vi "Motion Profile Tester.vi"() -> ()   [LabVIEW 2015]
uses:
  <vilib>/Rock Robotics/WPI/CAN/TalonSRX/WPI_CANTalonSRX_MotionProfileTrajectoryPt.ctl
  <vilib>/Rock Robotics/WPI/CAN/TalonSRX/WPI_CANTalonSRX_APIControlMode.ctl
  <vilib>/Rock Robotics/WPI/CAN/TalonSRX/WPI_CANTalonSRX_APIFeedbackSelect.ctl
  Support Code/Team900-VIs/OnButton/OnButtonSingle.vi
  <vilib>/Rock Robotics/WPI/MotorControl/WPI_MotorControlOpenCANTalonSRX.vi
panel:
  out "Motor values while Running Profile":cluster{dbl[], dbl[]}[](graph)
  out "Applied Throttle while Running Profile":cluster{dbl[], dbl[]}(graph)
  in  "Run at 100% Power and Graph":bool
  in  "Abort":bool
  in  "Generate, Load, and Run Profile":bool
  in  "Run Profile":bool
  in  "Load Profile":bool
  in  "Generate Profile and Clear Points":bool
  out "Generated Profile":cluster{dbl[], dbl[]}[](graph)
  in  "Mode":T1(ring)
  in  "Motion Profile Control Frame Rate":dbl
  in  "Rotations to Travel":dbl
  in  "Max Jerk (rotations/sec^3)":dbl
  in  "Max Acceleration (rotations/sec^2)":dbl
  in  "Max Speed (rotations/sec)":dbl
  # "If applied throttle exceeds about .95 at any point in the execution of the profile either max speed acceleration, or jerk must be lowered. If it goes below .8 except at the very beginning or end either max speed, acceleration, or jerk  should be increased. (These numbers are for profiles which are supposed to be completed as quickly as possible. In contexts where the priority is on other things such as reducing the amount of force or jerk acting on a gearbox other metrics must be used.)"
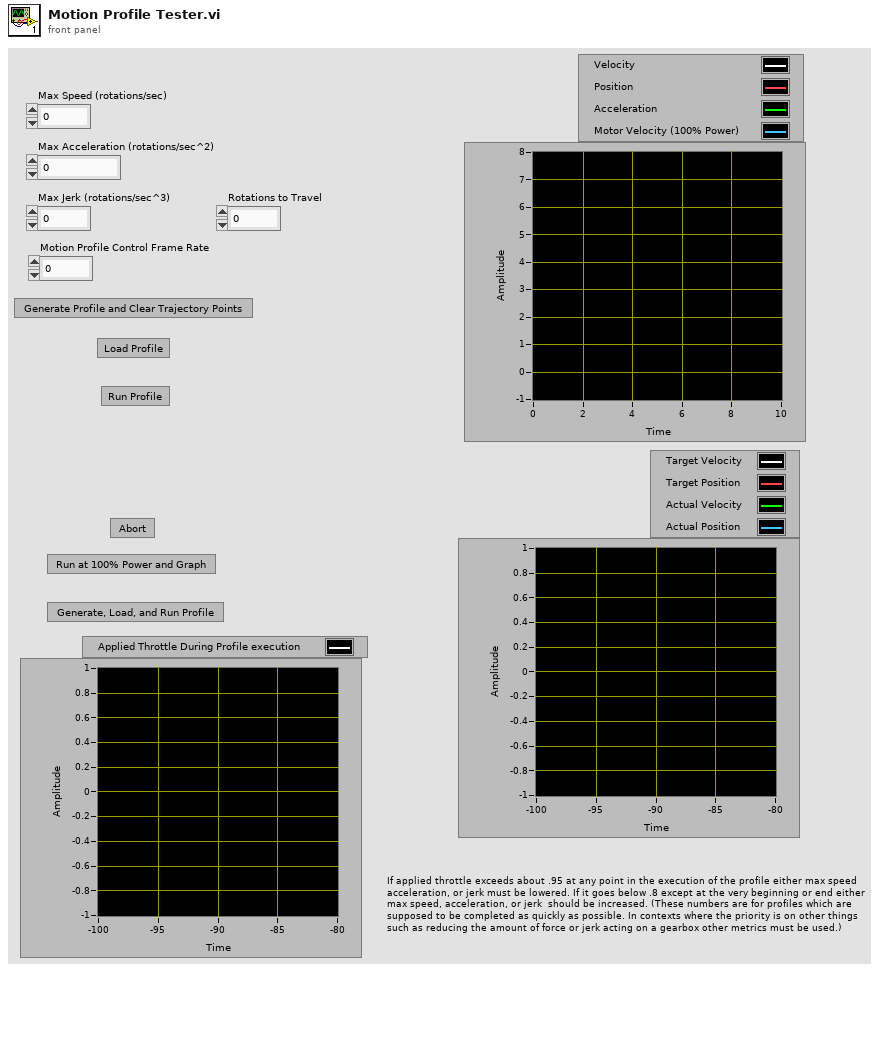
[diagram p1: front panel]
types:
  T1 = enum16{"Nothing", "Generate Profile and Clear", "Load Data to Motor", "Run Profile", "Run at 100% power and log"}
  T2 = typedef "WPI_CANTalonSRX_APIFeedbackSelect.ctl" = enum16{"Digital Quadrature Encoder", "Analog Potentiometer", "Analog Encoder", "Count on Quad-A (Rising-Edge)", "Count on Quad-A (Falling-Edge)", "CTR Magnetic Enc (Absolute)", "CTR Magnetic Enc (Relative)", "Pulse Width"}
  T3 = typedef "WPI_CANTalonSRX_APIControlMode.ctl" = enum8{"Percent VBus", "Speed", "Position", "Slave", "Unchanged / Invalid", "Voltage Compensation", "Current", "Motion Profile"}
  T4 = typedef "WPI_MotorControlDeviceRef.ctl" = cluster{"DeviceStatus":errorcluster, "Type":T5, "PWM":cluster{"PWM Channel":T6, "DeadBand":T7}, "CAN":cluster{"Device Number":u8, "Control Mode":T8, "Semaphore":T9, "Max Vout":dbl, "TalonSRX Control Mode":T3}, "Invert":bool}
  T5 = typedef "WPI_MotorControlType.ctl" = enum16{"PWM", "CAN", "CANTalonSRX"}
  T6 = typedef "FPGA_DIOPWMChannel.ctl" = enum8{"PWM 0", "PWM 1", "PWM 2", "PWM 3", "PWM 4", "PWM 5", "PWM 6", "PWM 7", "PWM 8", "PWM 9", "PWM MXP 0", "PWM MXP 1", "PWM MXP 2", "PWM MXP 3", "PWM MXP 4", "PWM MXP 5", "PWM MXP 6", "PWM MXP 7", "PWM MXP 8", "PWM MXP 9", "Invalid"}
  T7 = typedef "WPI_PWMDeadband.ctl" = cluster{"Name":string, "maxPositivePwm":i32, "minPositivePwm":i32, "centerPwm":i32, "maxNegativePwm":i32, "minNegativePwm":i32, "angularRange":u16}
  T8 = typedef "WPI_CANJaguar_ControlMode.ctl" = enum8{"Percent VBus", "Current", "Speed", "Position", "Voltage"}
  T9 = typedef "Semaphore RefNum" = refnum<k1>
  T10 = typedef "WPI_CANTalonSRX_MotionProfileTrajectoryPt.ctl" = cluster{"Duration Ms":u8, "Velocity":dbl, "Position":dbl, "Profile Slot Select":u8, "Is Last":bool, "Velocity Only":bool, "Zero Position":bool, "Compress Code":u8, "Same Velocity":i32, "Delta Position":i32, "Count":u8}
  T11 = enum16{"Nothing", "Generate Profile and Clear", "Load Data to Motor", "Run Profile"}
  T12 = enum16{"Nothing", "Generate Profile and Clear", "Load Data to Motor", "Run Profile", "Run at 100% power and log"}[]
  T13 = typedef "WPI_CANTalonSRX_GlobalStatus.ctl" = cluster{"Applied Throttle":dbl, "Module Enabled":bool, "CAN Error":errorcluster, "Closed Loop Error":dbl, "Forward Limit Switch Closed":bool, "Reverse Limit Switch Closed":bool, "Sensor Position":dbl, "Sensor Velocity":dbl, "Current":dbl, "Sticky Fault - Over Temp":bool, "Sticky Fault - Under Voltage":bool, "Sticky Fault - Forward Limit":bool, "Sticky Fault - Reverse Limit":bool, "Sticky Fault - Forward Soft Limit":bool, "Sticky Fault - Reverse Soft Limit":bool, "Brake is Enabled":bool, "Encoder Position":dbl, "Encoder Velocity":dbl, "Encoder Index Count":dbl, "Encoder A Pin State":bool, "Encoder B Pin State":bool, "Encoder Index Pin State":bool, "Analog In":dbl, "Analog In Velocity":dbl, "Temperature (C)":dbl, "Battery Voltage":dbl, "Control 5 Is Supported":bool, "Current Profile Slot Select":dbl, "Pos Div 8":bool, "Vel Div 4":bool, "Pulse Width Position":i32, "Pulse Width Velocity":i32, "Pulse Width Rise To Rise (us)":i32, "Pulse Width Rise To Fall (us)":i32, "Mot Prof Active Is Under Run":bool, "Mot Prof Active Has Under Run":bool, "Mot Prof Active Is Last":bool, "Mot Prof Active Velocity Only":bool, "Mot Prof Active Is Valid":bool, "Mot Prof Buffer Is Full":bool, "Mot Prof Active Profile Slot Select":i32, "Mot Prof NextID":i32, "Mot Prof Count":i32, "Mot Prof Active Velocity":dbl, "Mot Prof Active Position":dbl, "Mot Prof Output Enable":i32}
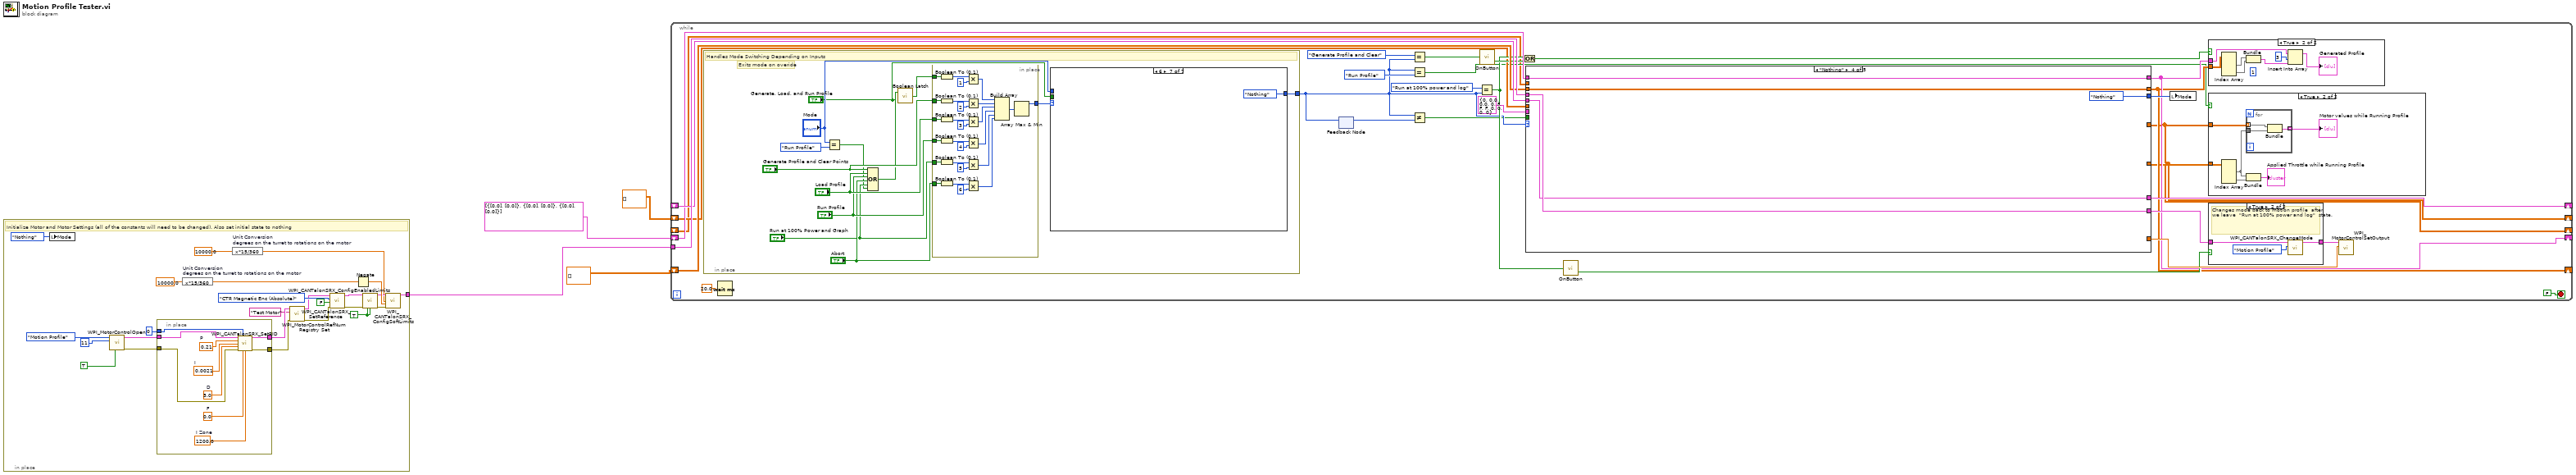
[diagram p0: block diagram]
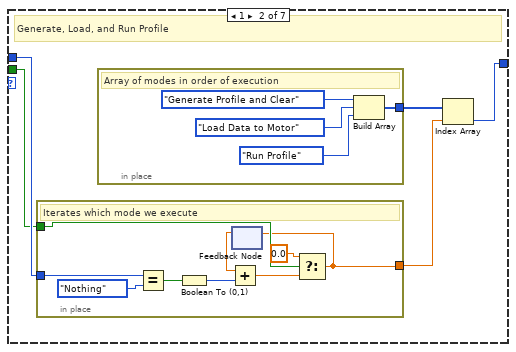
[diagram p6: hidden frame]
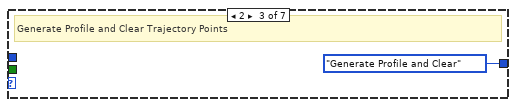
[diagram p7: hidden frame]
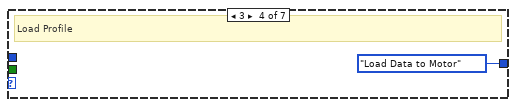
[diagram p8: hidden frame]
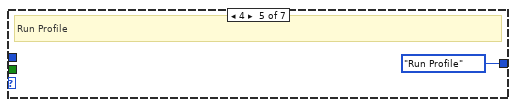
[diagram p9: hidden frame]
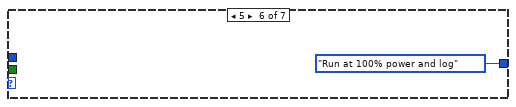
[diagram p10: hidden frame]
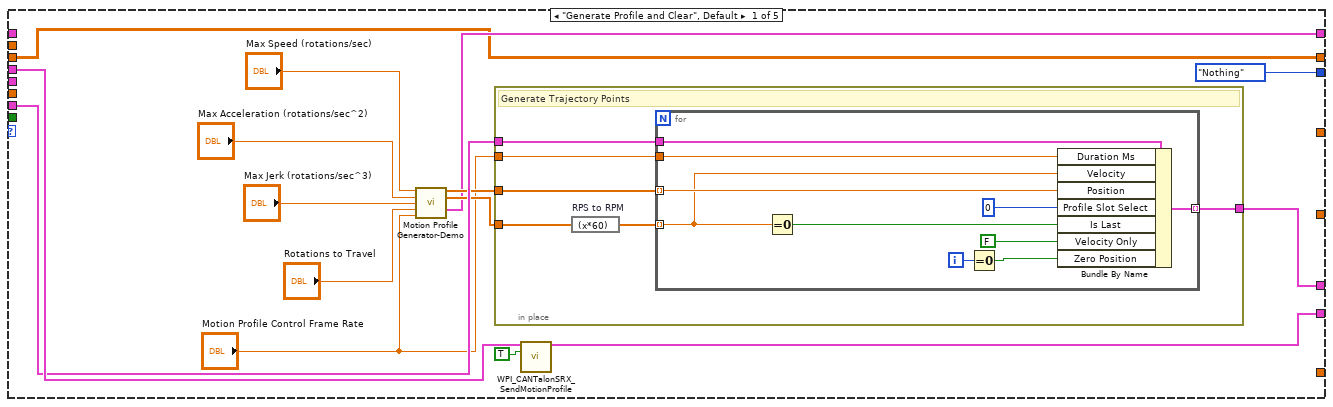
[diagram p11: hidden frame]
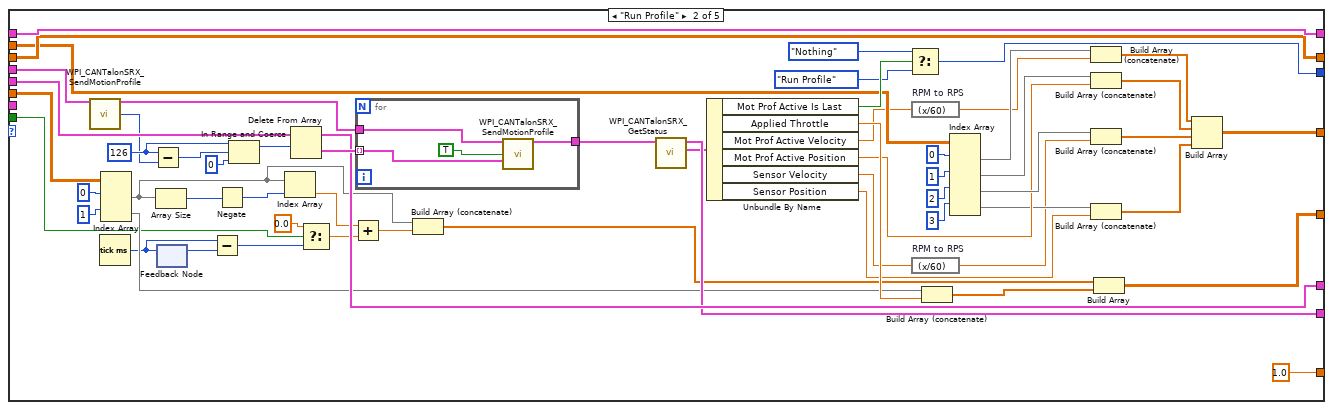
[diagram p12: hidden frame]
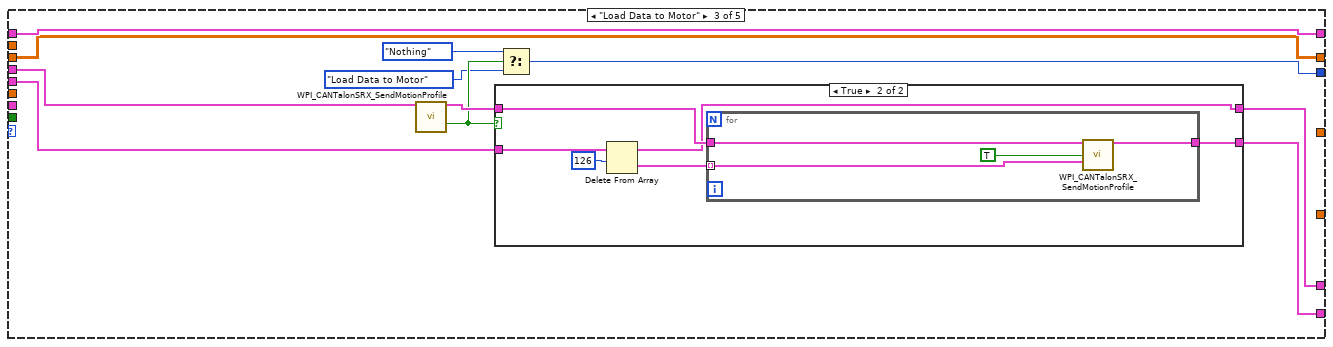
[diagram p13: hidden frame]
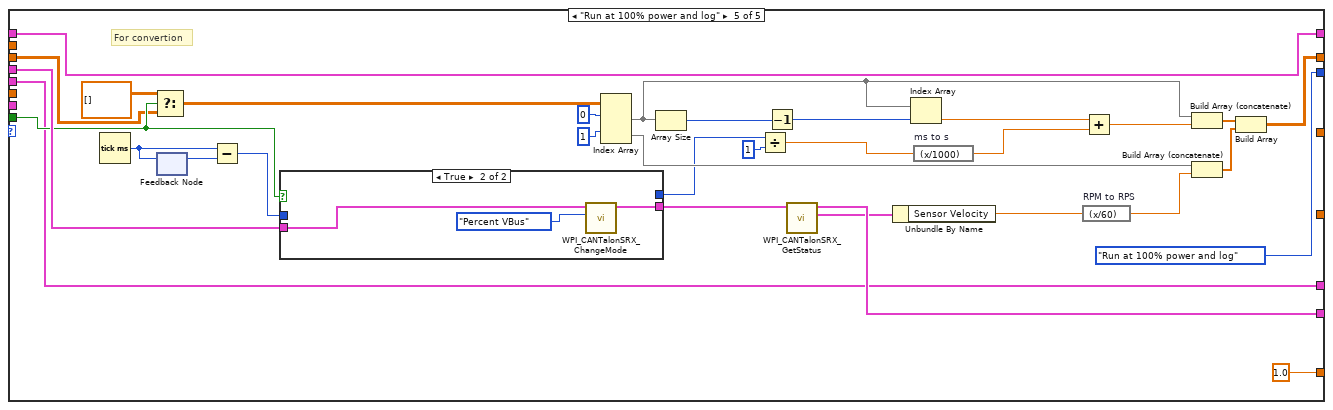
[diagram p15: hidden frame]
diagram:
  n1 = in-place {
    in-place-border: [w23] -> w4
    w19 = TRUE ("Forward Soft Limit Enable")
    # "Initialize Motor and Motor Settings (all of the constants will need to be changed). Also set initial state to nothing"
    n2 = local write "Mode"(T1."Nothing" ("Mode")) -> ()
    n3 = call-poly <vilib>:"WPI_MotorControlOpen.vi"("Invert"=TRUE, "Device Number"=11, "Control Mode"=WPI_CANTalonSRX_APIControlMode."Motion Profile") -> ("error out"=w26:errorcluster, "MotorControlDeviceRef"=w27:T4)  [unwired: 7 in]
    n4 = in-place {
      in-place-border: w27 -> [w39]
      in-place-border: w26 -> [w38]
      in-place-border: [w30] -> w10
      in-place-border: [w31] -> w12
      in-place-border: u8 0 ("Parameter Slot") -> [w32]
      w33 = 1200.0  # I Zone
      w34 = 0.0  # F
      w35 = 3.0  # D
      w36 = 0.0021  # I
      w37 = 0.21  # P
      n5 = call <vilib>:"WPI_CANTalonSRX_SetPID.vi"("CAN Talon SRX Ref"=w39, "Parameter Slot"=w32, "P"=w37, "I"=w36, "D"=w35, "error in (no error)"=w38, "F"=w34, "I Zone"=w33) -> ("CAN Talon SRX Ref"=w31:T4, "error out"=w30:errorcluster)  [unwired: 6 in]
    }
    n6 = expression code="x*15/360" "Unit Conversion\ndegrees on the turret to rotations on the motor"(10000.0 ("Forward Limit Position")) -> (w21:dbl)
    n7 = expression code="x*15/360" "Unit Conversion\ndegrees on the turret to rotations on the motor"(10000.0 ("Forward Limit Position")) -> (w13:dbl)
    n8 = call <vilib>:"WPI_MotorControlRefNum Registry Set.vi"("error in (no error)"=w10, "refnum name"="Test Motor", "MotorControlDevRef"=w12) -> ("error out"=w9:errorcluster, "MotorControlDevRef"=w11:T4)  [unwired: 7 in]
    n9 = call <vilib>:"WPI_CANTalonSRX_SetReference.vi"("error in (no error)"=w9, "Reverse Feedback Sensor"=FALSE, "Feedback Reference"=WPI_CANTalonSRX_APIFeedbackSelect."CTR Magnetic Enc (Absolute)", "CAN Talon SRX Ref"=w11) -> ("error out"=w6:errorcluster, "CAN Talon SRX Ref"=w7:T4)  [unwired: 6 in]
    n10 = Negate(x=w21) -> (-x=w20:dbl)
    n11 = call <vilib>:"WPI_CANTalonSRX_ConfigEnabledLimits.vi"("CAN Talon SRX Ref"=w7, "error in (no error)"=w6, "Forward Soft Limit Enable"=w19, "Reverse Soft Limit Enable"=w19) -> ("CAN Talon SRX Ref"=w17:T4, "error out"=w18:errorcluster)  [unwired: 10 in]
    n12 = call <vilib>:"WPI_CANTalonSRX_ConfigSoftLimits.vi"("CAN Talon SRX Ref"=w17, "Forward Limit Position"=w13, "Reverse Limit Position"=w20, "error in (no error)"=w18) -> ("CAN Talon SRX Ref"=w23:T4)  [unwired: 10 in, 1 out]
  }
  n13 = while {
    tunnel: w4 -> [w69]
    shift-right: [w67] -> _
    shift-left: _ -> [w64]
    shift-right: [w54] -> _
    shift-left: cluster{dbl[], dbl[]}[] [{[0.0], [0.0]}, {[0.0], [0.0]}, {[0.0], [0.0]}] ("XY Graph") -> [w56]
    shift-right: [w53] -> _
    shift-left: dbl[][] [] -> [w55]
    shift-right: [w45] -> _
    shift-left: dbl[][] [] -> [w48]
    shift-right: [w43] -> _
    shift-left: _ -> [w44]
    stop <- FALSE stop-if-true
    n14 = in-place {
      in-place-border: [w101] -> w42
      # "Exits mode on overide"
      # "Handles Mode Switching Depending on Inputs"
      n15 = Equal?(x="Mode", y=T11."Run Profile") -> (x = y?=w92:bool)
      n16 = Compound Arithmetic op=OR("Generate Profile and Clear Points", "Load Profile", "Run Profile", "Abort", "Run at 100% Power and Graph", w92) -> (w91:bool)
      n17 = call "Boolean Latch.vi"("Input"="Generate, Load, and Run Profile", "Reset"=w91) -> ("Output"=w98:bool)
      n18 = in-place {
        in-place-border: "Generate Profile and Clear Points" -> [w128]
        in-place-border: "Load Profile" -> [w123]
        in-place-border: w98 -> [w121]
        in-place-border: "Run Profile" -> [w119]
        in-place-border: [w117] -> w99
        in-place-border: "Abort" -> [w108]
        in-place-border: "Run at 100% Power and Graph" -> [w105]
        n19 = Boolean To (0,1)(Boolean=w121) -> (0, 1=w115:i16)
        n20 = Boolean To (0,1)(Boolean=w128) -> (0, 1=w127:i16)
        n21 = Boolean To (0,1)(Boolean=w123) -> (0, 1=w125:i16)
        n22 = Boolean To (0,1)(Boolean=w119) -> (0, 1=w116:i16)
        n23 = Boolean To (0,1)(Boolean=w105) -> (0, 1=w104:i16)
        n24 = Boolean To (0,1)(Boolean=w108) -> (0, 1=w107:i16)
        n25 = Multiply(x=w115, y=i16 1) -> (x*y=w112:i16)
        n26 = Multiply(x=w127, y=i16 2) -> (x*y=w111:i16)
        n27 = Multiply(x=w125, y=i16 3) -> (x*y=w110:i16)
        n28 = Multiply(x=w116, y=i16 4) -> (x*y=w109:i16)
        n29 = Multiply(x=w104, y=i16 5) -> (x*y=w103:i16)
        n30 = Multiply(x=w107, y=i16 6) -> (x*y=w106:i16)
        n31 = Build Array(w112, w111, w110, w109, w103, w106) -> (w118:i16[])
        n32 = Array Max & Min(array=w118) -> (max value=w117:i16)  [unwired: 3 out]
      }
      n33 = case shown="6" w99 {
        tunnel: [w129 w130 T1."Generate Profile and Clear" ("Mode") T1."Load Data to Motor" ("Mode") T1."Run Profile" ("Mode") T1."Run at 100% power and log" ("Mode") T1."Nothing" ("Mode")] -> w101
        tunnel: "Mode" -> [w129 w134 _ _ _ _ _]
        tunnel: "Generate, Load, and Run Profile" -> [_ w133 _ _ _ _ _]
        frame 0, Default {
          # "Carry last operation"
        }
        frame 1 {
          # "Generate, Load, and Run Profile"
          n34 = in-place {
            in-place-border: w134 -> [w143]
            in-place-border: w133 -> [w138]
            in-place-border: [w135] -> w131
            # "Iterates which mode we execute"
            n35 = Equal?(x=w143, y=T11."Nothing") -> (x = y?=w141:bool)
            n36 = Boolean To (0,1)(Boolean=w141) -> (0, 1=w140:i16)
            n37 = feedback #1() -> (w139:dbl)  [unwired: 1 in]
            n38 = Add(x=w139, y=w140) -> (x+y=w136:dbl)
            n39 = Select(t=0.0, s=w138, f=w136) -> (s? t:f=w135:dbl)
            n40 = feedback-in #1(w135) -> ()
          }
          n41 = in-place {
            in-place-border: [w147] -> w132
            # "Array of modes in order of execution"
            n42 = Build Array(T1."Generate Profile and Clear" ("Mode"), T1."Load Data to Motor" ("Mode"), T1."Run Profile" ("Mode")) -> (w147:T12)
          }
          n43 = Index Array(array=w132, index=w131) -> (element=w130:T1)
        }
        frame 2 {
          # "Generate Profile and Clear Trajectory Points"
        }
        frame 3 {
          # "Load Profile"
        }
        frame 4 {
          # "Run Profile"
        }
        frame 5 {
        }
        frame 6 {
        }
      }
    }
    n44 = Wait (ms)(milliseconds to wait=20.0) -> ()  [unwired: 1 out]
    n45 = feedback-in #2(w42) -> ()
    n46 = feedback #2() -> (w41:T1)  [unwired: 1 in]
    n47 = Equal?(x=T1."Generate Profile and Clear", y=w42) -> (x = y?=w52:bool)
    n48 = Equal?(x=w42, y=T1."Run Profile") -> (x = y?=w46:bool)
    n49 = Not Equal?(x=w42, y=w41) -> (x != y?=w40:bool)
    n50 = Equal?(x=T1."Run at 100% power and log", y=w42) -> (x = y?=w49:bool)
    n51 = call-poly "OnButton.vi"("Input"=w52) -> ("Released"=w51:bool)  [unwired: 1 out]
    n52 = Or(x=w49, y=w51) -> (x .or. y?=w50:bool)
    n53 = case shown="\"Nothing\"" w42 {
      tunnel: w69 -> [w163 w240 w256 w274 w306]
      tunnel: T10 {"Duration Ms"=0, "Velocity"=0.0, "Position"=0.0, "Profile Slot Select"=0, "Is Last"=FALSE, "Velocity Only"=FALSE, "Zero Position"=FALSE, "Compress Code"=0, "Same Velocity"=0, "Delta Position"=0, "Count"=0} ("New Point") -> [w162 _ _ _ _]
      tunnel: [w159 w234 w254 w273 w276] -> w67
      tunnel: [T1."Nothing" ("Mode") w231 w252 T1."Nothing" ("Mode") T1."Run at 100% power and log" ("Mode")] -> w65
      tunnel: w64 -> [_ w241 w257 w273 w276]
      tunnel: [w158 w233 w251 w274 w302] -> w58
      tunnel: [_ 1.0 _ _ 1.0] -> w62
      tunnel: w40 -> [_ w195 _ _ w293]
      tunnel: [w155 w224 w247 w270 w295] -> w53
      tunnel: [w156 w225 w248 w271 w301] -> w54
      tunnel: w56 -> [_ w225 w248 w271 w301]
      tunnel: w55 -> [w155 w224 w247 w270 w292]
      tunnel: w48 -> [_ w223 _ _ _]
      tunnel: [_ w219 _ _ _] -> w45
      tunnel: w44 -> [_ w211 _ _ _]
      tunnel: [_ w198 _ _ _] -> w43
      frame "Generate Profile and Clear", Default {
        n54 = call "Motion Profile Generator-Demo.vi"("Max Speed (rotations/sec)"="Max Speed (rotations/sec)", "Max Acceleration (rotations/sec^2)"="Max Acceleration (rotations/sec^2)", "Max Jerk (rotations/sec^3)"="Max Jerk (rotations/sec^3)", "Rotations to Travel"="Rotations to Travel", "Motion Profile Control Frame Rate"="Motion Profile Control Frame Rate") -> ("Position rotations"=w160:dbl[], "velocity rotations/sec"=w161:dbl[], "XY Graph"=w156:cluster{dbl[], dbl[]}[])  [unwired: 7 in, 1 out]
        n55 = in-place {
          in-place-border: w162 -> [w173]
          in-place-border: w161 -> [w169]
          in-place-border: w160 -> [w172]
          in-place-border: "Motion Profile Control Frame Rate" -> [w171]
          in-place-border: [w170] -> w159
          # "Generate Trajectory Points"
          n56 = expression code="(x*60)" "RPS to RPM"(w169) -> (w168:dbl[])
          n57 = for {
            tunnel: w173 -> [w183]
            tunnel: w168 -> [w179] mode=indexing
            tunnel: w172 -> [w181] mode=indexing
            tunnel: w171 -> [w180]
            tunnel: [w174] -> w170 mode=indexing
            i -> [w176]
            n58 = Equal To 0?(x=w179) -> (x = 0?=w178:bool)
            n59 = Equal To 0?(x=w176) -> (x = 0?=w175:bool)
            n60 = Bundle By Name(cluster=w183, "Duration Ms"=w180, "Velocity"=w179, "Position"=w181, "Profile Slot Select"=u8 0, "Is Last"=w178, "Velocity Only"=FALSE, "Zero Position"=w175) -> (w174:T10)
          }
        }
        n61 = call <vilib>:"WPI_CANTalonSRX_SendMotionProfile.vi"("CAN Talon SRX Ref"=w163, "Clear"=TRUE) -> ("CAN Talon SRX Ref Out"=w158:T4)  [unwired: 10 in, 3 out]
      }
      frame "Run Profile" {
        w238 = u32 126 ("x")
        n62 = call <vilib>:"WPI_CANTalonSRX_SendMotionProfile.vi"("CAN Talon SRX Ref"=w240) -> ("CAN Talon SRX Ref Out"=w228:T4, "Count"=w229:u32)  [unwired: 11 in, 2 out]
        n63 = Tick Count (ms)() -> (millisecond timer value=w197:u32)
        n64 = Index Array(array=w223, index (row) #1=0 ("index (row)"), index (row) #2=1 ("index (row)")) -> (element #1=w190:dbl[], element #2=w221:dbl[])  [unwired: 2 in]
        n65 = Subtract(x=w238, y=w229) -> (x-y=w239:u32)
        n66 = Array Size(array=w190) -> (size(s)=w192:i32)
        n67 = feedback #3() -> (w196:u32)  [unwired: 1 in]
        n68 = feedback-in #3(w197) -> ()
        n69 = Subtract(x=w197, y=w196) -> (x-y=w193:u32)
        n70 = Negate(x=w192) -> (-x=w191:i32)
        n71 = In Range and Coerce(upper limit=w238, x=w239, lower limit=u32 0) -> (coerced(x)=w235:u32)  [unwired: 1 out]
        n72 = Index Array(array=w190, index=w191) -> (element=w189:dbl)
        n73 = Delete From Array(array=w241, length=w235) -> (deleted portion=w236:T10[], array with subset deleted=w234:T10[])  [unwired: 1 in]
        n74 = Select(t=0.0, s=w195, f=w193) -> (s? t:f=w188:dbl)
        n75 = Add(x=w189, y=w188) -> (x+y=w220:dbl)
        n76 = for {
          tunnel: w236 -> [w246] mode=indexing
          tunnel: w228 -> [w244]
          tunnel: [w243] -> w216
          n77 = call <vilib>:"WPI_CANTalonSRX_SendMotionProfile.vi"("CAN Talon SRX Ref"=w244, "Push"=TRUE, "New Point"=w246) -> ("CAN Talon SRX Ref Out"=w243:T4)  [unwired: 9 in, 3 out]
        }
        n78 = Build Array (concatenate)(w190, w220) -> (w218:dbl[])
        n79 = call <vilib>:"WPI_CANTalonSRX_GetStatus.vi"("CAN Talon SRX Ref"=w216) -> ("Talon SRX Status"=w232:T13, "CAN Talon SRX Ref"=w233:T4)  [unwired: 8 in, 1 out]
        n80 = Unbundle By Name(w232) -> ("Mot Prof Active Is Last"=w230:bool, "Applied Throttle"=w222:dbl, "Mot Prof Active Velocity"=w187:dbl, "Mot Prof Active Position"=w204:dbl, "Sensor Velocity"=w185:dbl, "Sensor Position"=w202:dbl)
        n81 = Select(t=T1."Nothing" ("Mode"), s=w230, f=T1."Run Profile" ("Mode")) -> (s? t:f=w231:T1)
        n82 = expression code="(x/60)" "RPM to RPS"(w187) -> (w186:dbl)
        n83 = expression code="(x/60)" "RPM to RPS"(w185) -> (w184:dbl)
        n84 = Build Array (concatenate)(w221, w222) -> (w217:dbl[])
        n85 = Index Array(array=w211, index (row) #1=0 ("index (row)"), index (row) #2=1 ("index (row)"), index (row) #3=2 ("index (row)"), index (row) #4=3 ("index (row)")) -> (element #1=w214:dbl[], element #2=w215:dbl[], element #3=w205:dbl[], element #4=w200:dbl[])  [unwired: 4 in]
        n86 = Build Array (concatenate)(w214, w186) -> (w213:dbl[])
        n87 = Build Array (concatenate)(w215, w204) -> (w212:dbl[])
        n88 = Build Array (concatenate)(w205, w184) -> (w203:dbl[])
        n89 = Build Array (concatenate)(w200, w202) -> (w199:dbl[])
        n90 = Build Array(w218, w217) -> (w219:dbl[][])
        n91 = Build Array(w213, w212, w203, w199) -> (w198:dbl[][])
      }
      frame "Load Data to Motor" {
        n92 = call <vilib>:"WPI_CANTalonSRX_SendMotionProfile.vi"("CAN Talon SRX Ref"=w256) -> ("CAN Talon SRX Ref Out"=w255:T4, "Ready For Next"=w253:bool)  [unwired: 11 in, 2 out]
        n93 = case shown="True" w253 {
          tunnel: w257 -> [w259 w265]
          tunnel: w255 -> [w258 w262]
          tunnel: [w259 w261] -> w254
          tunnel: [w258 w260] -> w251
          frame False {
          }
          frame True {
            n94 = Delete From Array(array=w265, length=126) -> (deleted portion=w263:T10[], array with subset deleted=w261:T10[])  [unwired: 1 in]
            n95 = for {
              tunnel: w263 -> [w269] mode=indexing
              tunnel: w262 -> [w268]
              tunnel: [w267] -> w260
              n96 = call <vilib>:"WPI_CANTalonSRX_SendMotionProfile.vi"("CAN Talon SRX Ref"=w268, "Push"=TRUE, "New Point"=w269) -> ("CAN Talon SRX Ref Out"=w267:T4)  [unwired: 9 in, 3 out]
            }
          }
        }
        n97 = Select(t=T1."Nothing" ("Mode"), s=w253, f=T1."Load Data to Motor" ("Mode")) -> (s? t:f=w252:T1)
      }
      frame "Nothing" {
      }
      frame "Run at 100% power and log" {
        # "For convertion"
        n98 = Tick Count (ms)() -> (millisecond timer value=w280:u32)
        n99 = Select(t=dbl[][] [], s=w293, f=w292) -> (s? t:f=w290:dbl[][])
        n100 = feedback #4() -> (w279:u32)  [unwired: 1 in]
        n101 = feedback-in #4(w280) -> ()
        n102 = Subtract(x=w280, y=w279) -> (x-y=w278:u32)
        n103 = case shown="True" w293 {
          tunnel: w306 -> [w308 w311]
          tunnel: [w308 w310] -> w303
          tunnel: [w307 _] -> w287
          tunnel: w278 -> [w307 _]
          frame False {
          }
          frame True {
            n104 = call <vilib>:"WPI_CANTalonSRX_ChangeMode.vi"("Control Mode"=WPI_CANTalonSRX_APIControlMode."Percent VBus", "CAN Talon SRX Ref"=w311) -> ("CAN Talon SRX Ref"=w310:T4)  [unwired: 8 in, 1 out]
          }
        }
        n105 = Index Array(array=w290, index (row) #1=0 ("index (row)"), index (row) #2=1 ("index (row)")) -> (element #1=w283:dbl[], element #2=w298:dbl[])  [unwired: 2 in]
        n106 = Array Size(array=w283) -> (size(s)=w284:i32)
        n107 = Divide(x=w287, y=u32 1) -> (x/y=w285:dbl)
        n108 = Decrement(x=w284) -> (x-1=w282:i32)
        n109 = call <vilib>:"WPI_CANTalonSRX_GetStatus.vi"("CAN Talon SRX Ref"=w303) -> ("Talon SRX Status"=w277:T13, "CAN Talon SRX Ref"=w302:T4)  [unwired: 8 in, 1 out]
        n110 = Unbundle By Name(w277) -> ("Sensor Velocity"=w275:dbl)
        n111 = Index Array(array=w283, index=w282) -> (element=w281:dbl)
        n112 = expression code="(x/1000)" "ms to s"(w285) -> (w289:dbl)
        n113 = expression code="(x/60)" "RPM to RPS"(w275) -> (w294:dbl)
        n114 = Add(x=w281, y=w289) -> (x+y=w288:dbl)
        n115 = Build Array (concatenate)(w283, w288) -> (w297:dbl[])
        n116 = Build Array (concatenate)(w298, w294) -> (w296:dbl[])
        n117 = Build Array(w297, w296) -> (w295:dbl[][])
      }
    }
    n118 = call-poly "OnButton.vi"("Input"=w49) -> ("Released"=w60:bool)  [unwired: 1 out]
    n119 = local write "Mode"(w65) -> ()
    n120 = case shown="True" w50 {
      tunnel: w54 -> [_ w85]
      tunnel: w53 -> [_ w82]
      frame False {
      }
      frame True {
        (unwired) 1 ("index (row)")
        n121 = Index Array(array=w82) -> (element #1=w81:dbl[], element #2=w80:dbl[])  [unwired: 4 in]
        n122 = Bundle(w81, w80) -> (w79:cluster{dbl[], dbl[]})  [unwired: 1 in]
        n123 = Insert Into Array(array=w85, index=3, new element=w79) -> (→"Generated Profile":cluster{dbl[], dbl[]}[])
      }
    }
    n124 = case shown="True" w46 {
      tunnel: w45 -> [_ w75]
      tunnel: w43 -> [_ w72]
      frame False {
      }
      frame True {
        n125 = Index Array(array=w75) -> (element #1=w71:dbl[], element #2=w74:dbl[])  [unwired: 4 in]
        n126 = for {
          tunnel: w72 -> [w78] mode=indexing
          tunnel: w71 -> [w77]
          tunnel: [w76] -> w70 mode=indexing
          n127 = Bundle(w78, w77) -> (w76:cluster{dbl[], dbl[]})  [unwired: 1 in]
        }
        "Motor values while Running Profile" <- w70
        n128 = Bundle(w71, w74) -> (→"Applied Throttle while Running Profile":cluster{dbl[], dbl[]})  [unwired: 1 in]
      }
    }
    n129 = case shown="True" w60 {
      tunnel: w58 -> [w86 w89]
      tunnel: [w86 w88] -> w59
      frame False {
      }
      frame True {
        # "Changes mode back to motion profile  after we leave  \"Run at 100% power and log\"  state."
        n130 = call <vilib>:"WPI_CANTalonSRX_ChangeMode.vi"("Control Mode"=WPI_CANTalonSRX_APIControlMode."Motion Profile", "CAN Talon SRX Ref"=w89) -> ("CAN Talon SRX Ref"=w88:T4)  [unwired: 8 in, 1 out]
      }
    }
    n131 = call <vilib>:"WPI_MotorControlSetOutput.vi"("Output"=w62, "MotorControlDevRef"=w59) -> ()  [unwired: 7 in, 3 out]
  }
